vi "Get IP Resolver.vi"(8 "error in (no error)":errorcluster, 11 "Node in":refnum<class "Node Config.lvclass">) -> (0 "error out":errorcluster, 2 "IP Resolver":refnum<class "IP Resolver.lvclass">, 3 "Node out":refnum<class "Node Config.lvclass">)   [LabVIEW 2020, in "VolatusConfig.lvlib" / "Node Config.lvclass"]
uses:
  Node Config.lvclass
  C:/dev/lv20CE/relink/lv-volatus/VolatusConfig/VolatusConfigElement/VolatusConfigElement.lvclass
  VolatusConfigElement/VolatusConfigElement.lvclass/VolatusConfigElement.ctl
  VolatusConfigElement/Element.vi
  Node Config.lvclass/Node Config.ctl
  VolatusConfigElement/VolatusConfigElement.lvclass
  lv-cdm/CDM-Config/Config Element/Config Element.lvclass
  lv-vecto/Vecto/IP Resolver/IP Resolver.lvclass
  C:/dev/lv20CE/relink/lv-volatus/VolatusConfig/Node/Node Config.lvclass
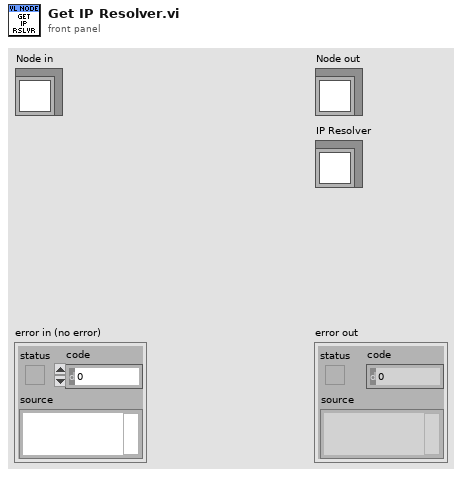
[diagram p1: front panel]
types:
  T1 = typedef "CDM-Config.lvlib/Value Type.ctl" = enum16{"String", "Number", "Bool", "Object", "Array"}
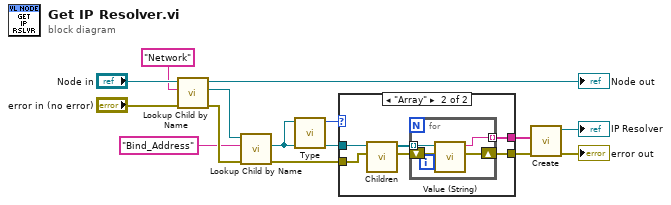
[diagram p0: block diagram]
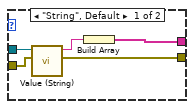
[diagram p2: hidden frame]
diagram:
  n1 = call "Lookup Child by Name.vi"("error in (no error)"="error in (no error)", "Child Name"="Network", "VolatusConfigElement in"="Node in") -> ("error out"=w9:errorcluster, "Child"=w10:refnum<class "Config Element.lvclass">, "VolatusConfigElement out"=→"Node out":refnum<class "Node Config.lvclass">)  [unwired: 5 in, 1 out]
  n2 = call "Lookup Child by Name.vi"("error in (no error)"=w9, "Name"="Bind_Address", "Config Element in"=w10) -> ("error out"=w5:errorcluster, "Child"=w6:refnum<class "Config Element.lvclass">)  [unwired: 5 in, 2 out]
  n3 = call "Type.vi"("Config Element in"=w6) -> ("Value Type"=w7:T1)  [unwired: 9 in, 1 out]
  n4 = case shown="\"Array\"" w7 {
    tunnel: w6 -> [w19 w25]
    tunnel: w5 -> [w18 w23]
    tunnel: [w17 w21] -> w4
    tunnel: [w15 w20] -> w3
    frame "String", Default {
      n5 = call "Value (String).vi"("error in (no error)"=w18, "Config Element in"=w19) -> ("error out"=w15:errorcluster, "String Value"=w16:string)  [unwired: 8 in]
      n6 = Build Array(w16) -> (w17:string[])
    }
    frame "Array" {
      n7 = call "Children.vi"("error in (no error)"=w23, "Config Element in"=w25) -> ("error out"=w22:errorcluster, "Elements"=w24:refnum<class "Config Element.lvclass">[])  [unwired: 8 in]
      n8 = for {
        tunnel: w24 -> [w29] mode=indexing
        shift-right: [w27] -> w20
        shift-left: w22 -> [w28]
        tunnel: [w26] -> w21 mode=indexing
        n9 = call "Value (String).vi"("error in (no error)"=w28, "Config Element in"=w29) -> ("error out"=w27:errorcluster, "String Value"=w26:string)  [unwired: 8 in]
      }
    }
  }
  n10 = call "Create.vi"("error in (no error)"=w3, "Bindings"=w4) -> ("error out"=→"error out":errorcluster, "IP Resolver"=→"IP Resolver":refnum<class "IP Resolver.lvclass">)  [unwired: 8 in]
